vi "Trim Sensitivity.vi"(0 "TSM context":T2, 1 "Program OTP?(F)":bool, 5 "Target Sensitivity (dBV)":dbl format="%#_13g", 7 "Trim Method":T1) -> (15 "error out":errorcluster)   [LabVIEW 2020]
doc: "Trims sensitivity of the DUT by adjusting the Gain and Vbias values using Trim protocol"
uses:
  <vilib>/NI_TestStand_SemiconductorModule/NI_TestStand_Semiconductor_Module.lvlibp/PinMap/General/SemiconductorModuleContext.ctl
  SubVIs/Trim Method Enum.ctl
  Common/Instrument Control/Digital/TSM/TSM SSC Digital.ctl
  <vilib>/NI_TestStand_SemiconductorModule/NI_TestStand_Semiconductor_Module.lvlibp/PinMap/Digital Pattern/PinQueryContext/DigitalPatternPinQueryContext.lvclass
  Common/Instrument Control/Digital/SSC Digital/SSC Digital.ctl
  Common/Instrument Control/DCPower/TSM/TSM SSC DCPower.ctl
  <vilib>/NI_TestStand_SemiconductorModule/NI_TestStand_Semiconductor_Module.lvlibp/PinMap/PinQueryContext/MultiplePinMultipleSessionQueryContext/MultiplePinMultipleSessionQueryContext.lvclass
  Common/Instrument Control/DCPower/SSC DCPower/SSC DCPower.ctl
  Common/Instrument Control/Shared SubVIs/TSM Pin Abstraction/TSM Pin Information.ctl
  Common/Instrument Control/Shared SubVIs/TSM Pin Abstraction/TSM Pin Type Identifier.ctl
  Common/Instrument Control/Shared SubVIs/TSM Pin Abstraction/TSM Expanded Pin Information.ctl
  Common/DUT Control/Typedefs/DUT Read Commands.ctl
  <vilib>/NI_TestStand_SemiconductorModule/NI_TestStand_Semiconductor_Module.lvlibp/PinMap/TagProvider/TSM_PublishedDataId.ctl
  <vilib>/NI_TestStand_SemiconductorModule/NI_TestStand_Semiconductor_Module.lvlibp/PinMap/TagProvider/TSM_InputDataId.ctl
  Common/DUT Control/Typedefs/DUT Write Commands.ctl
  <instrlib>/niDigital/niDigital.llb/niDigital Write Static Pin State.ctl
  354e2fd9-1388-4924-804e-e9490b2eeb0b.vi
  46ecd2fd-2f0c-4e5f-b596-d218653973fe.vi
  c53558f2-5030-41db-922a-32af9ad26e5f.vi
  354e2fd9-1388-4924-804e-e9490b2eeb0b.vi/71683651-cbc5-46e0-8522-40ce4dc1e9ef.vi
  354e2fd9-1388-4924-804e-e9490b2eeb0b.vi/5048e37d-0f89-4c33-89a7-b3c71e857334.vi
  354e2fd9-1388-4924-804e-e9490b2eeb0b.vi/0bdf4848-63d7-49b9-a33f-cfc1e4c0521b.vi
  354e2fd9-1388-4924-804e-e9490b2eeb0b.vi/b8e335d8-4854-4718-8e9f-88d363955659.vi
  Common/Instrument Control/Digital/TSM/TSM SSC Digital N Pins To M Sessions.vi
  <vilib>/NI_TestStand_SemiconductorModule/NI_TestStand_Semiconductor_Module.lvlibp/PinMap/Input Data/GetInputDataDouble.vi
  Common/Instrument Control/DCPower/SSC DCPower/Source/SSC DCPower Configure Output Enabled.vi
  Common/Instrument Control/DCPower/SSC DCPower/Source/Constant Voltage/SSC DCPower Force Voltage Array Symmetric Limits.vi
  <vilib>/NI_TestStand_SemiconductorModule/NI_TestStand_Semiconductor_Module.lvlibp/PinMap/Relay Driver/ControlRelay(s).vi
  <vilib>/NI_TestStand_SemiconductorModule/NI_TestStand_Semiconductor_Module.lvlibp/PinMap/Relay Driver/ApplyRelayConfiguration.vi
  <vilib>/NI_TestStand_SemiconductorModule/NI_TestStand_Semiconductor_Module.lvlibp/PinMap/General/Publish/PublishDataBoolFunctionalTest.vi
  <vilib>/NI_TestStand_SemiconductorModule/NI_TestStand_Semiconductor_Module.lvlibp/PinMap/General/Publish/PublishDataDoubleFunctionalTest.vi
  Common/Instrument Control/Digital/SSC Digital/Static/SSC Digital Write Static.vi
  <vilib>/NI_TestStand_SemiconductorModule/NI_TestStand_Semiconductor_Module.lvlibp
  Common/Instrument Control/Digital/SSC Digital/Pin Levels and Timing/SSC Digital Single Level Selection.ctl
panel:
  out "PreTrimOTP Input":dbl[](array[numeric])
  out "Trim Sens":dbl[](array[numeric])
  out "PreTrim Sens":dbl[](array[numeric])
  out "Trim Write + Echo":u8[][](array[numeric])
  out "Pre Trim Read":u8[][](array[numeric])
  # "<Gain>       <Vbias>  <Mode>   <OTP>"
  # "<Gain><Vbias><Mode><OTP><OTP Echo>"
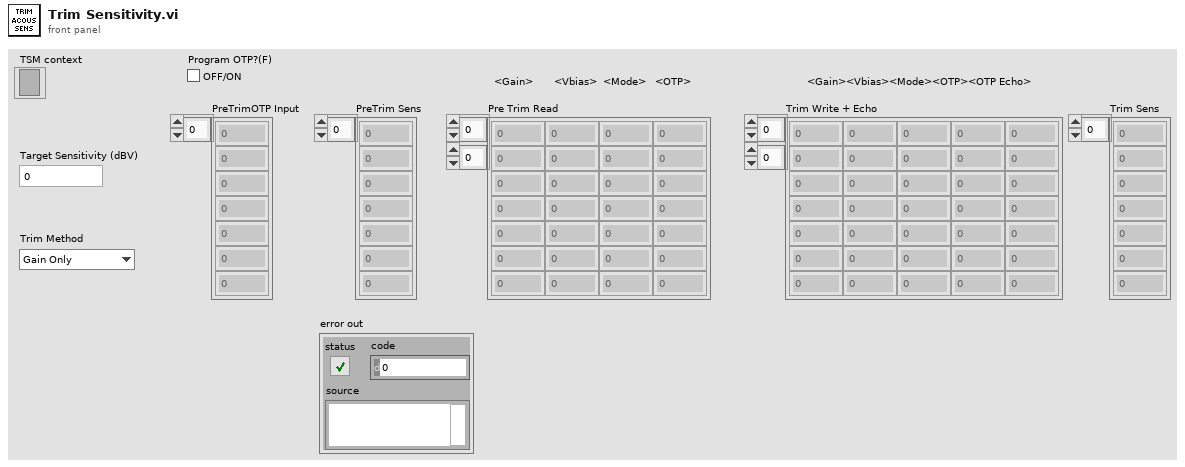
[diagram p1: front panel]
types:
  T1 = typedef "Trim Method Enum.ctl" = enum16{"Gain Only", "Gain then Vbias", "Gain Vbias Combo"}
  T2 = typedef "NI_TestStand_Semiconductor_Module.lvlibp/SemiconductorModuleContext.ctl" = refnum<k7>
  T3 = typedef "TSM SSC Digital.ctl" = cluster{"Pin Query Context":refnum<class "DigitalPatternPinQueryContext.lvclass">, "SSC":T4[], "Site Numbers":i32[], "Pins":tag[]}
  T4 = typedef "SSC Digital.ctl" = cluster{"Session":refnum<k15>, "Channel List":string, "Site List":string}
  T5 = typedef "TSM SSC DCPower.ctl" = cluster{"Pin Query Context":refnum<class "MultiplePinMultipleSessionQueryContext.lvclass">, "SSC":T6[], "Site Numbers":i32[], "Pins":T7[], "Pins Expanded":T9[]}
  T6 = typedef "SSC DCPower.ctl" = cluster{"Session":refnum<k15>, "Chan":string, "Channel List":string}
  T7 = typedef "TSM Pin Information.ctl" = cluster{"Pin":tag, "Type":T8, "Count":i32}
  T8 = typedef "TSM Pin Type Identifier.ctl" = enum8{"DUT Pin", "System Pin", "Pin Group", "Not Determined"}
  T9 = typedef "TSM Expanded Pin Information.ctl" = cluster{"Pin":tag, "Type":T8, "Index":i32}
  T10 = cluster{"OTP Pins":T3, "SMU_VDD_MERGED":T5, "PreTrim Sensitivity":dbl[], "PreTrimOTP":u8[], "HSD_OUT+":T3}
  T11 = typedef "SSC Digital Single Level Selection.ctl" = enum16{"Vil", "Vih", "Vol", "Voh", "Vterm", "Iol", "Ioh", "Vcom"}
  T12 = typedef "NI_TestStand_Semiconductor_Module.lvlibp/TSM_InputDataId.ctl" = tag
  T13 = typedef "NI_TestStand_Semiconductor_Module.lvlibp/TSM_PublishedDataId.ctl" = tag
  T14 = typedef "DUT Read Commands.ctl" = enum16{"Read Reg and Timeout", "Read OTP and Timeout"}
  T15 = typedef "DUT Write Commands.ctl" = enum16{"Write Reg and Timeout", "Write Reg and Nmode Cmd", "Program OTP"}
  T16 = typedef "niDigital Write Static Pin State.ctl" = u8
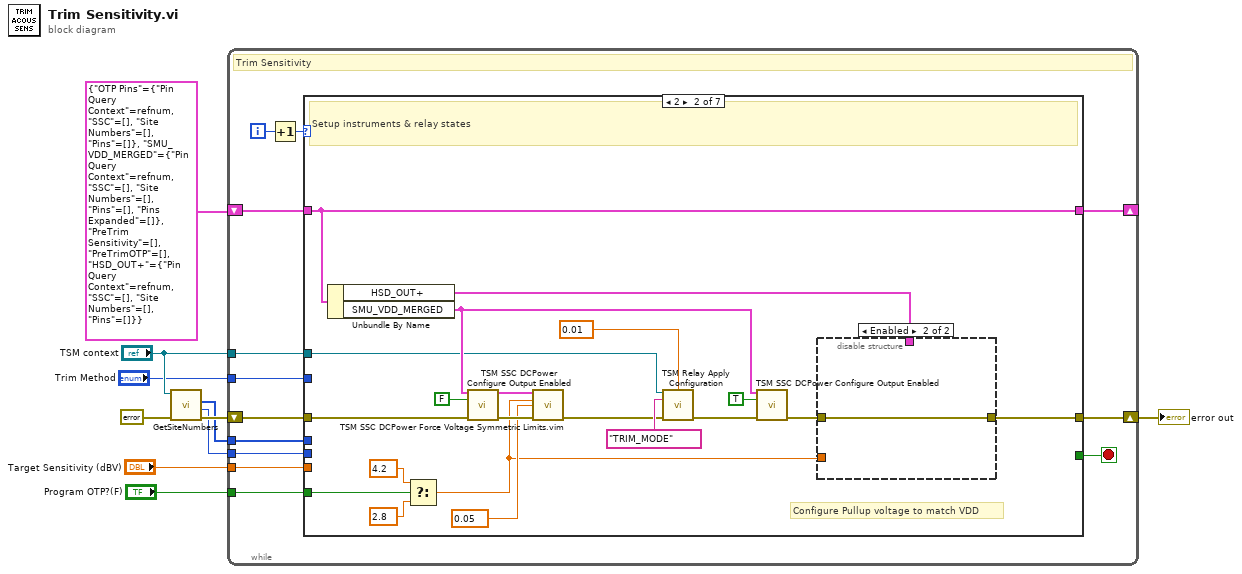
[diagram p0: block diagram]
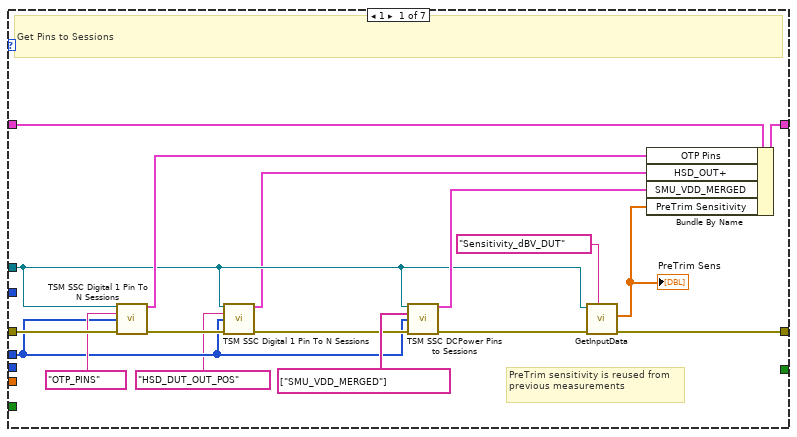
[diagram p2: hidden frame]
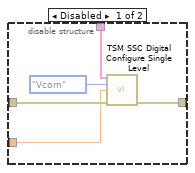
[diagram p3: hidden frame]
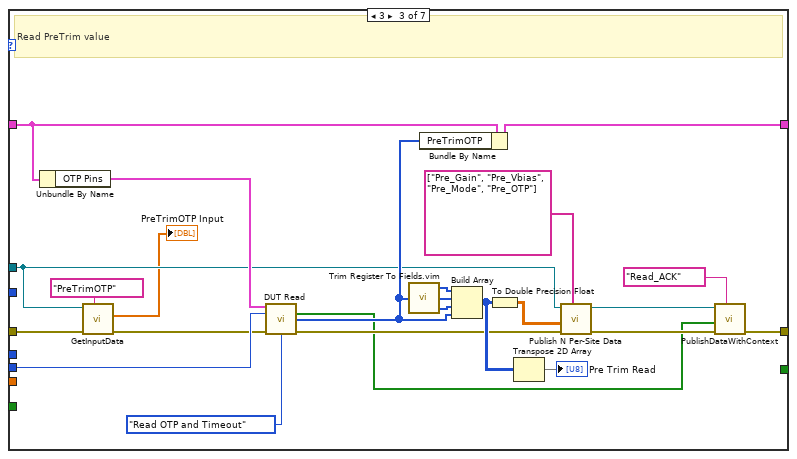
[diagram p4: hidden frame]
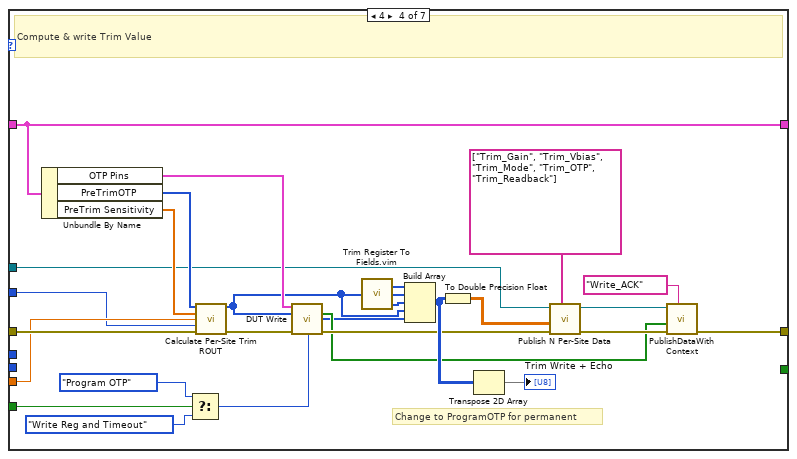
[diagram p5: hidden frame]
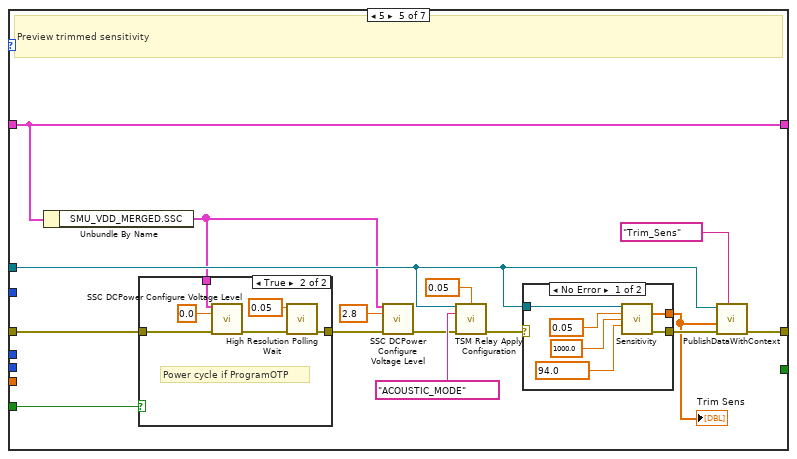
[diagram p6: hidden frame]
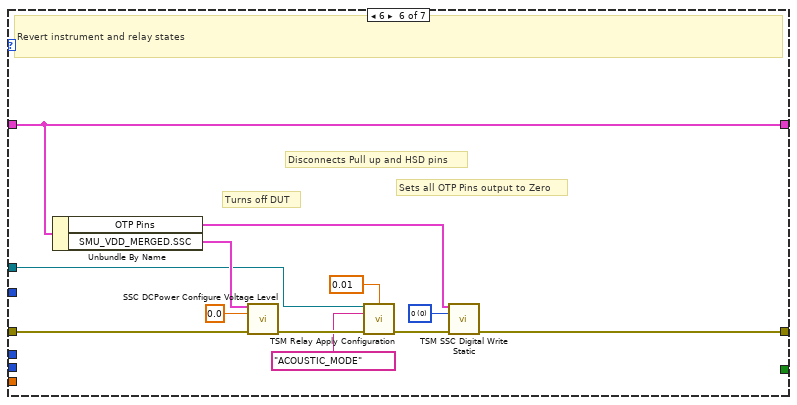
[diagram p9: hidden frame]
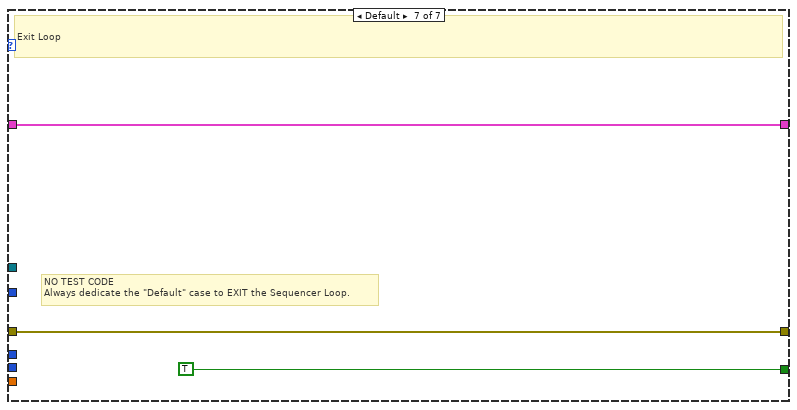
[diagram p10: hidden frame]
diagram:
  n1 = call <vilib>:"GetSiteNumbers.vi"("error in (no error)"=errorcluster {"status"=FALSE, "code"=0, "source"=""} ("error in"), "Semiconductor Module Context"="TSM context") -> ("error out"=w7:errorcluster, "Number Of Sites"=w3:i32, "Site Numbers"=w5:i32[])  [unwired: 6 in, 1 out]
  n2 = while {
    shift-right: [w21] -> w10
    shift-left: w7 -> [w22]
    tunnel: "TSM context" -> [w19]
    shift-right: [w16] -> _
    shift-left: T10 {"OTP Pins"={"Pin Query Context"=refnum, "SSC"=[], "Site Numbers"=[], "Pins"=[]}, "SMU_VDD_MERGED"={"Pin Query Context"=refnum, "SSC"=[], "Site Numbers"=[], "Pins"=[], "Pins Expanded"=[]}, "PreTrim Sensitivity"=[], "PreTrimOTP"=[], "HSD_OUT+"={"Pin Query Context"=refnum, "SSC"=[], "Site Numbers"=[], "Pins"=[]}} -> [w17]
    tunnel: w5 -> [w15]
    tunnel: "Target Sensitivity (dBV)" -> [w14]
    tunnel: w3 -> [w13]
    tunnel: "Program OTP?(F)" -> [w12]
    tunnel: "Trim Method" -> [w11]
    i -> [w23]
    stop <- w18 stop-if-true
    # "Trim Sensitivity"
    n3 = Increment(x=w23) -> (x+1=w20:i32)
    n4 = case shown="2" w20 {
      tunnel: [w32 w46 w75 w97 w126 w148 w161] -> w21
      tunnel: w22 -> [w40 w60 w89 w118 w122 w159 w161]
      tunnel: w19 -> [w28 w48 w70 w103 w124 w153 _]
      tunnel: [_ _ _ _ _ _ TRUE] -> w18
      tunnel: w17 -> [w39 w56 w87 w115 w128 w156 w160]
      tunnel: [w37 w56 w78 w115 w128 w156 w160] -> w16
      tunnel: w15 -> [w26 _ _ _ _ _ _]
      tunnel: w14 -> [_ _ _ w116 _ _ _]
      tunnel: w13 -> [_ _ w88 _ _ _ _]
      tunnel: w12 -> [_ w41 _ w101 w119 _ _]
      tunnel: w11 -> [_ _ _ w92 _ _ _]
      frame 1 {
        # "PreTrim sensitivity is reused from previous measurements"
        # "Get Pins to Sessions"
        n5 = call "TSM SSC Digital 1 Pin To N Sessions.vi"("TSM context"=w28, "Pin"=tag "OTP_PINS", "Site Numbers"=w26, "error in"=w40) -> ("Digital TSM Out"=w36:T3, "error out"=w29:errorcluster)  [unwired: 10 in]
        n6 = call "TSM SSC Digital 1 Pin To N Sessions.vi"("TSM context"=w28, "Pin"=tag "HSD_DUT_OUT_POS", "Site Numbers"=w26, "error in"=w29) -> ("Digital TSM Out"=w24:T3, "error out"=w27:errorcluster)  [unwired: 10 in]
        n7 = call "TSM SSC DCPower Pins to Sessions.vi"("TSM context"=w28, "Pins"=tag[] ["SMU_VDD_MERGED"], "Site Numbers"=w26, "error in"=w27) -> ("DCPower TSM Out"=w34:T5, "error out"=w31:errorcluster)  [unwired: 10 in]
        n8 = call-poly <vilib>:"GetInputData.vi"("Input Data Id"=tag "Sensitivity_dBV_DUT", "error in (no error)"=w31, "Semiconductor Module Context"=w28) -> ("error out"=w32:errorcluster, "Data Out"=w30:dbl[])  [unwired: 6 in, 1 out]
        "PreTrim Sens" <- w30
        n9 = Bundle By Name(cluster=w39, "OTP Pins"=w36, "HSD_OUT+"=w24, "SMU_VDD_MERGED"=w34, "PreTrim Sensitivity"=w30) -> (w37:T10)
      }
      frame 2 {
        # "Configure Pullup voltage to match VDD"
        # "Setup instruments & relay states"
        n10 = Unbundle By Name(w56) -> ("HSD_OUT+"=w45:T3, "SMU_VDD_MERGED"=w52:T5)
        n11 = Select(t=4.2 ("Voltage Level (V)"), s=w41, f=2.8 ("Voltage Level (V)")) -> (s? t:f=w44:dbl)
        n12 = call "TSM SSC DCPower Configure Output Enabled.vi"("DCPower TSM in"=w52, "Output Enabled"=FALSE, "error in"=w60) -> ("DCPower TSM out"=w55:T5, "error out"=w59:errorcluster)  [unwired: 11 in]
        n13 = call "TSM SSC DCPower Force Voltage Symmetric Limits.vim"("DCPower TSM in"=w55, "Voltage Level (V)"=w44, "Current Limit (A)"=0.05, "error in"=w59) -> ("error out"=w49:errorcluster)  [unwired: 10 in, 1 out]
        n14 = call "TSM Relay Apply Configuration.vi"("TSM Context"=w48, "Settling Time (0s)"=0.01, "Relay Configuration"=tag "TRIM_MODE", "error in (no error)"=w49) -> ("error out"=w51:errorcluster)  [unwired: 11 in]
        n15 = call "TSM SSC DCPower Configure Output Enabled.vi"("DCPower TSM in"=w52, "Output Enabled"=TRUE, "error in"=w51) -> ("error out"=w58:errorcluster)  [unwired: 11 in, 1 out]
        n16 = disable-structure shown="Enabled" {
          disable-tunnel: w58 -> [w65 w66]
          disable-tunnel: [w64 w66] -> w46
          disable-tunnel: w44 -> [w62 _]
          disable-tunnel: w45 -> [w61 _]
          frame Disabled {
            n17 = call "TSM SSC Digital Configure Single Level.vi"("Digital TSM In"=w61, "Level Type to Set"=SSC_Digital_Single_Level_Selection."Vcom", "Setting"=w62, "error in"=w65) -> ("error out"=w64:errorcluster)  [unwired: 10 in, 1 out]
          }
          frame Enabled {
          }
        }
      }
      frame 3 {
        # "Read PreTrim value"
        n18 = Unbundle By Name(w87) -> ("OTP Pins"=w86:T3)
        n19 = call-poly <vilib>:"GetInputData.vi"("Input Data Id"=T12 "PreTrimOTP", "error in (no error)"=w89, "Semiconductor Module Context"=w70) -> ("error out"=w68:errorcluster, "Data Out"=→"PreTrimOTP Input":dbl[])  [unwired: 6 in, 1 out]
        n20 = call "DUT Read.vi"("Digital TSM In"=w86, "Number Of Sites"=w88, "error in (no error)"=w68, "Operation"=DUT_Read_Commands."Read OTP and Timeout") -> ("Per-Site Pass"=w73:bool[], "Per Site Read Data"=w77:u8[], "error out"=w80:errorcluster)  [unwired: 8 in, 1 out]
        n21 = call "Trim Register To Fields.vim"("ROUT"=w77) -> ("Mode"=w83:u8[], "Vbias"=w84:u8[], "Gain"=w85:u8[])  [unwired: 2 in]
        n22 = Bundle By Name(cluster=w87, "PreTrimOTP"=w77) -> (w78:T10)
        n23 = Build Array(w85, w84, w83, w77) -> (w82:u8[][])
        n24 = To Double Precision Float(number=w82) -> (double precision float=w79:dbl[][])
        n25 = Transpose 2D Array(2D array=w82) -> (transposed array=→"Pre Trim Read":u8[][])
        n26 = call "Publish N Per-Site Data.vi"("Published Data Id"=tag[] ["Pre_Gain", "Pre_Vbias", "Pre_Mode", "Pre_OTP"], "error in (no error)"=w80, "Data In"=w79, "Semiconductor Module Context"=w70) -> ("error out"=w76:errorcluster, "Semiconductor Module Context Out"=w74:T2)  [unwired: 6 in]
        n27 = call-poly <vilib>:"PublishDataWithContext.vi"("Published Data Id"=T13 "Read_ACK", "error in (no error)"=w76, "Data In"=w73, "Semiconductor Module Context"=w74) -> ("error out"=w75:errorcluster)  [unwired: 6 in, 1 out]
      }
      frame 4 {
        # "Change to ProgramOTP for permanent"
        # "Compute & write Trim Value"
        n28 = Unbundle By Name(w115) -> ("OTP Pins"=w112:T3, "PreTrimOTP"=w114:u8[], "PreTrim Sensitivity"=w113:dbl[])
        n29 = Select(t=DUT_Write_Commands."Program OTP" ("Operation"), s=w101, f=DUT_Write_Commands."Write Reg and Timeout" ("Operation")) -> (s? t:f=w98:T15)
        n30 = call "Calculate Per-Site Trim ROUT.vi"("Per Site ROUT In"=w114, "Per-Site Cur Sensitivity(dBV)"=w113, "Target Sensitivity(dBV)"=w116, "Trim Method"=w92, "error in (no error)"=w118) -> ("Per Site ROUT Out"=w104:u8[], "error out"=w117:errorcluster)  [unwired: 8 in, 1 out]
        n31 = call "DUT Write.vi"("Digital TSM In"=w112, "Per Site Data In"=w104, "error in (no error)"=w117, "Operation"=w98) -> ("Per-Site Pass"=w96:bool[], "Per Site Data Out"=w94:u8[], "error out"=w106:errorcluster)  [unwired: 8 in, 1 out]
        n32 = call "Trim Register To Fields.vim"("ROUT"=w104) -> ("Mode"=w109:u8[], "Vbias"=w110:u8[], "Gain"=w111:u8[])  [unwired: 2 in]
        n33 = Build Array(w111, w110, w109, w104, w94) -> (w108:u8[][])
        n34 = To Double Precision Float(number=w108) -> (double precision float=w105:dbl[][])
        n35 = Transpose 2D Array(2D array=w108) -> (transposed array=→"Trim Write + Echo":u8[][])
        n36 = call "Publish N Per-Site Data.vi"("Published Data Id"=tag[] ["Trim_Gain", "Trim_Vbias", "Trim_Mode", "Trim_OTP", "Trim_Readback"], "error in (no error)"=w106, "Data In"=w105, "Semiconductor Module Context"=w103) -> ("error out"=w102:errorcluster, "Semiconductor Module Context Out"=w95:T2)  [unwired: 6 in]
        n37 = call-poly <vilib>:"PublishDataWithContext.vi"("Published Data Id"=T13 "Write_ACK", "error in (no error)"=w102, "Data In"=w96, "Semiconductor Module Context"=w95) -> ("error out"=w97:errorcluster)  [unwired: 6 in, 1 out]
      }
      frame 5 {
        # "Preview trimmed sensitivity"
        n38 = Unbundle By Name(w128) -> ("SMU_VDD_MERGED.SSC"=w120:T6[])
        n39 = case shown="True" w119 {
          tunnel: w122 -> [w134 w139]
          tunnel: [w134 w137] -> w121
          tunnel: w120 -> [_ w135]
          frame False {
          }
          frame True {
            # "Power cycle if ProgramOTP"
            n40 = call "SSC DCPower Configure Voltage Level.vi"("DCPower SSC in"=w135, "Voltage Level (V)"=0.0, "error in"=w139) -> ("error out"=w138:errorcluster)  [unwired: 11 in, 1 out]
            n41 = call <vilib>:"High Resolution Polling Wait.vi"("error in (no error)"=w138, "seconds to wait"=0.05) -> ("error out"=w137:errorcluster)  [unwired: 9 in]
          }
        }
        n42 = call "SSC DCPower Configure Voltage Level.vi"("DCPower SSC in"=w120, "Voltage Level (V)"=2.8, "error in"=w121) -> ("error out"=w129:errorcluster)  [unwired: 11 in, 1 out]
        n43 = call "TSM Relay Apply Configuration.vi"("TSM Context"=w124, "Settling Time (0s)"=0.05, "Relay Configuration"=tag "ACOUSTIC_MODE", "error in (no error)"=w129) -> ("error out"=w131:errorcluster)  [unwired: 11 in]
        n44 = case shown="No Error" w131 {
          selector: w131 -> [_ w147]
          tunnel: [w146 w147] -> w130
          tunnel: [w145 _] -> w125
          tunnel: w124 -> [w141 _]
          frame No Error {
            n45 = call "Sensitivity.vi"("TSM context"=w141, "Capture Duration (s)"=0.05, "Frequency"=1000.0, "dB SPL"=94.0) -> ("dB V"=w145:dbl[], "error out"=w146:errorcluster)  [unwired: 9 in, 1 out]
          }
          frame Error {
          }
        }
        "Trim Sens" <- w125
        n46 = call-poly <vilib>:"PublishDataWithContext.vi"("Published Data Id"=tag "Trim_Sens", "error in (no error)"=w130, "Data In"=w125, "Semiconductor Module Context"=w124) -> ("error out"=w126:errorcluster)  [unwired: 6 in, 1 out]
      }
      frame 6 {
        w151 = T16 0 items=["0"=0, "1"=1, "X"=5] ("State")
        # "Sets all OTP Pins output to Zero"
        # "Disconnects Pull up and HSD pins"
        # "Turns off DUT"
        # "Revert instrument and relay states"
        n47 = Unbundle By Name(w156) -> ("OTP Pins"=w150:T3, "SMU_VDD_MERGED.SSC"=w155:T6[])
        n48 = call "SSC DCPower Configure Voltage Level.vi"("DCPower SSC in"=w155, "Voltage Level (V)"=0.0, "error in"=w159) -> ("error out"=w158:errorcluster)  [unwired: 11 in, 1 out]
        n49 = call "TSM Relay Apply Configuration.vi"("TSM Context"=w153, "Settling Time (0s)"=0.01, "Relay Configuration"=tag "ACOUSTIC_MODE", "error in (no error)"=w158) -> ("error out"=w149:errorcluster)  [unwired: 11 in]
        n50 = call "TSM SSC Digital Write Static.vi"("Digital TSM in"=w150, "State"=w151, "error in"=w149) -> ("error out"=w148:errorcluster)  [unwired: 11 in, 1 out]
      }
      frame Default {
        # "NO TEST CODE\nAlways dedicate the \"Default\" case to EXIT the Sequencer Loop."
        # "Exit Loop"
      }
    }
  }
  "error out" <- w10
